vi "Runtime Dequeue and Execute Driver.vi"   [LabVIEW 2013]
types:
  T1 = typedef "Runtime Queue.ctl" = refnum<queue>
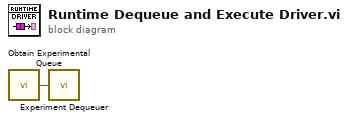
[diagram p0: block diagram]
diagram:
  n1 = call "Obtain Experimental Queue.vi"() -> ("Experimental Queue"=w1:T1)
  n2 = call "Experiment Dequeuer.vi"("Experiment Queue"=w1) -> ()
